vi "SIMULATION_SIM_Gyro_EXECUTE.vi"(6 "FPGA_Time_Seconds":dbl, 8 "error in (no error)":errorcluster) -> (0 "error out":errorcluster)   [LabVIEW 2019]
uses:
  Swerve_Drive_System/SWERVE_DRIVE_GLOBALS.vi
  SIMULATION_SIM_Globals.vi
  <vilib>/Rock Robotics/WPI/ThirdParty/JAS_Junk/TrajLib/Trajectory_Library.lvlib
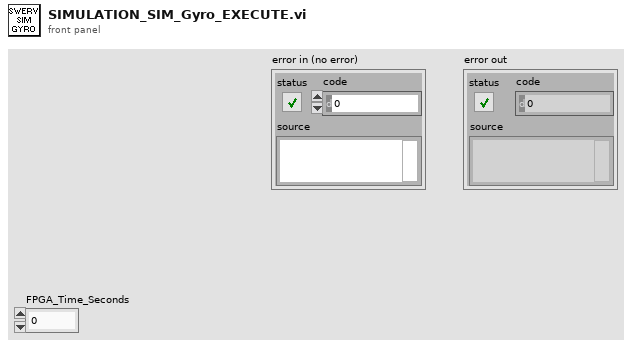
[diagram p1: front panel]
types:
  T1 = typedef "Trajectory_Library.lvlib/CHASSIS_SPEEDS.ctl" = cluster{"vX":dbl, "vY":dbl, "vOmega":dbl}
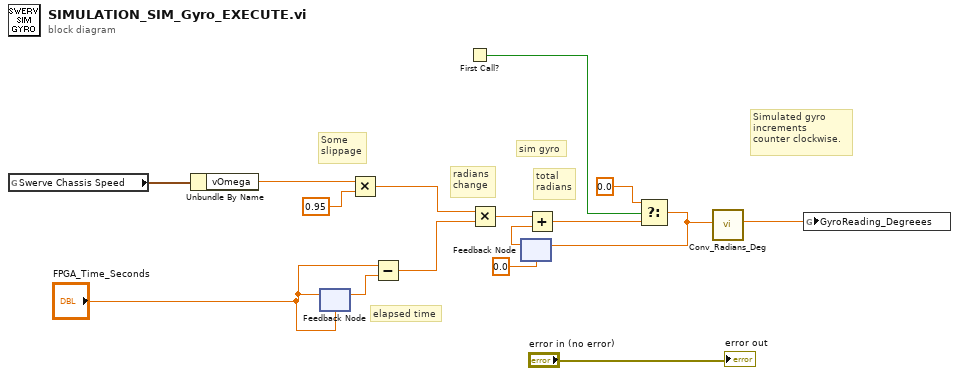
[diagram p0: block diagram]
diagram:
  # "Simulated gyro\nincrements\ncounter clockwise."
  # "Some \nslippage"
  # "elapsed time"
  # "total \nradians"
  # "radians \nchange"
  # "sim gyro"
  n1 = global read "SWERVE_DRIVE_GLOBALS.vi" "Swerve Chassis Speed"() -> (w16:T1)
  n2 = Unbundle By Name(w16) -> ("vOmega"=w15:dbl)
  n3 = feedback #1("FPGA_Time_Seconds") -> (w11:dbl)
  n4 = feedback-in #1("FPGA_Time_Seconds") -> ()
  n5 = Multiply(x=w15, y=0.95) -> (x*y=w9:dbl)
  n6 = Subtract(x="FPGA_Time_Seconds", y=w11) -> (x-y=w10:dbl)
  n7 = First Call?() -> (First Call?: T/F=w2:bool)
  n8 = Multiply(x=w9, y=w10) -> (x*y=w12:dbl)
  n9 = feedback #2(0.0) -> (w13:dbl)
  n10 = Add(x=w12, y=w13) -> (x+y=w4:dbl)
  n11 = Select(t=0.0, s=w2, f=w4) -> (s? t:f=w3:dbl)
  n12 = feedback-in #2(w3) -> ()
  n13 = call <vilib>:"Conv_Radians_Deg.vi"("Radians"=w3) -> ("Degrees"=w7:dbl)  [unwired: 10 in]
  n14 = global write "SIMULATION_SIM_Globals.vi" "GyroReading_Degreees"(w7) -> ()
  "error out" <- "error in (no error)"
